vi "SetZ_step.vi"(8 "错误输入（无错误）":errorcluster, 10 "step":i32, 11 "VISA资源名称":refnum<visa-resource-name>) -> (0 "错误输出":errorcluster, 3 "VISA资源名称输出":refnum<visa-resource-name>)   [LabVIEW 2018]
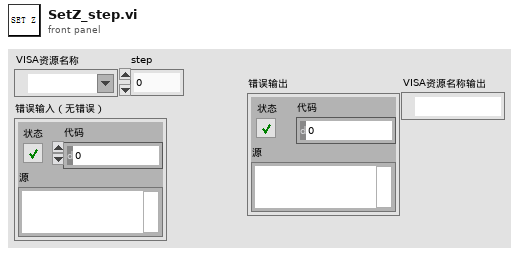
[diagram p1: front panel]
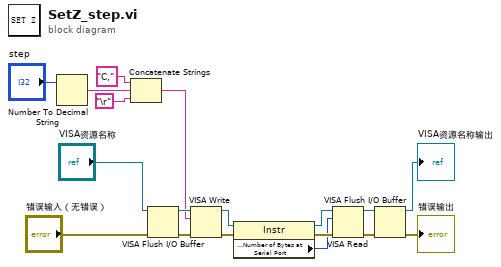
[diagram p0: block diagram]
diagram:
  n1 = Number To Decimal String(number="step") -> (decimal integer string=w6:string)  [unwired: 1 in]
  n2 = Concatenate Strings("C," ("字符串"), w6, "\r") -> (w8:string)
  n3 = VISA Flush I/O Buffer(VISA resource name="VISA资源名称", error in (no error)="错误输入（无错误）") -> (VISA resource name out=w10:refnum<visa-resource-name>, error out=w9:errorcluster)  [unwired: 1 in]
  n4 = VISA Write ("VISA写入")(VISA resource name=w10, write buffer=w8, error in (no error)=w9) -> (VISA resource name out=w16:refnum<visa-resource-name>, error out=w17:errorcluster)  [unwired: 1 out]
  n5 = property class="Instr"(reference=w16, error in=w17) -> (reference out=w15:refnum<visa-resource-name>, error out=w14:errorcluster, "Serial Settings:Number of Bytes at Serial Port"=w11:u32)
  n6 = VISA Read(VISA resource name=w15, byte count=w11, error in (no error)=w14) -> (VISA resource name out=w13:refnum<visa-resource-name>, error out=w12:errorcluster)  [unwired: 2 out]
  n7 = VISA Flush I/O Buffer(VISA resource name=w13, error in (no error)=w12) -> (VISA resource name out=→"VISA资源名称输出":refnum<visa-resource-name>, error out=→"错误输出":errorcluster)  [unwired: 1 in]
